vi "Write Template FN.vi"(8 "error in (no error)":errorcluster, 10 "Template FN":string, 11 "XLS in":refnum<class "XLS.lvclass">) -> (0 "error out":errorcluster, 3 "XLS out":refnum<class "XLS.lvclass">)   [LabVIEW 2017, in "Report_lib.lvlib" / "XLS.lvclass"]
uses:
  XLS.lvclass
  XLS.lvclass/XLS.ctl
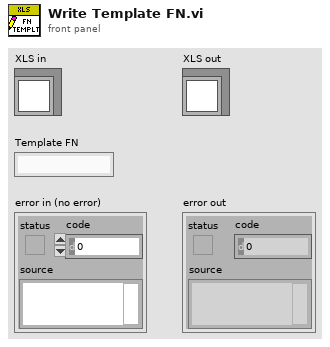
[diagram p1: front panel]
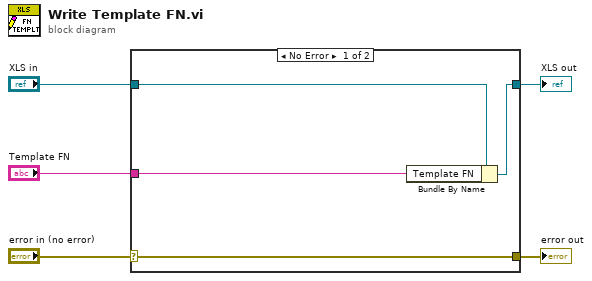
[diagram p0: block diagram]
diagram:
  n1 = case shown="No Error" "error in (no error)" {
    selector: "error in (no error)" -> [w9 w10]
    tunnel: [w9 w10] -> w4
    tunnel: [w7 w11] -> w2
    tunnel: "XLS in" -> [w8 w11]
    tunnel: "Template FN" -> [w6 _]
    frame No Error {
      n2 = Bundle By Name(cluster=w8, "Template FN"=w6) -> (w7:refnum<class "XLS.lvclass">)
    }
    frame Error {
    }
  }
  "error out" <- w4
  "XLS out" <- w2
